vi "move.vi"() -> ()   [LabVIEW 2011]
uses:
  <vilib>/express/express arith-compare/Formula/XNode/ExpressFormulaBlockNode.xnode
panel:
  out "Obs":string
  in  "Boolean":bool
  out "Numero Impar":dbl
  in  "Generar NUmero Par 2":bool
  in  "Generar NUmero Par":bool
  out "Numero par":dbl
  # "Usando eventos generar un numero par al presionar un generar\npar y generar un impar al presionar un numero imprar"
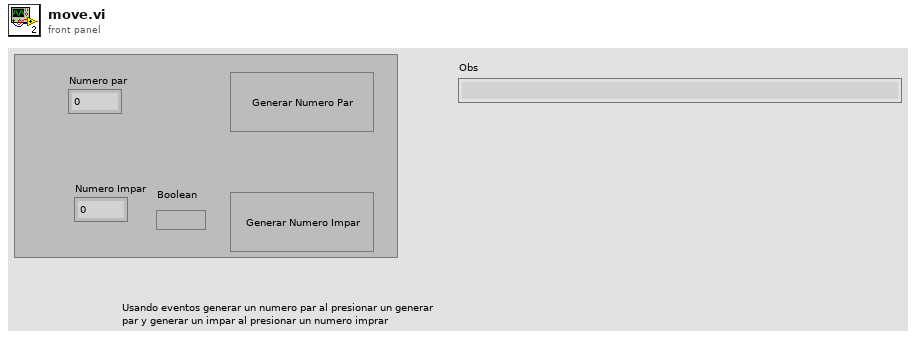
[diagram p1: front panel]
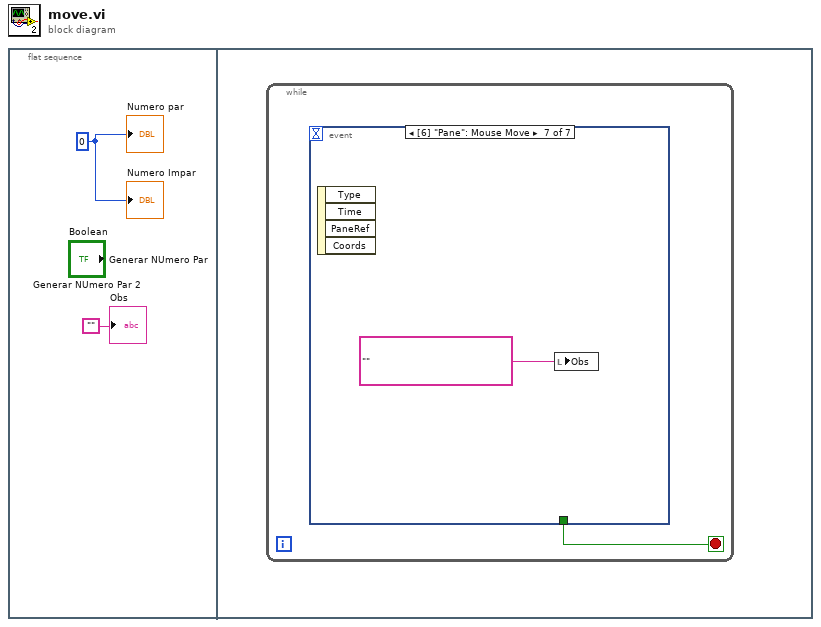
[diagram p0: block diagram]
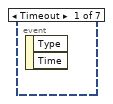
[diagram p2: hidden frame]
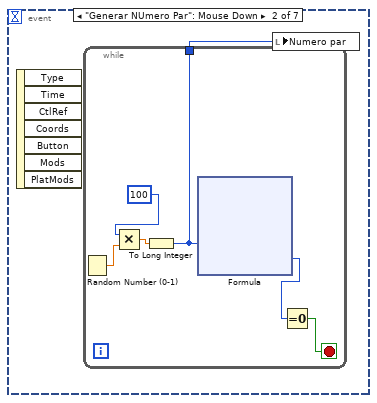
[diagram p3: hidden frame]
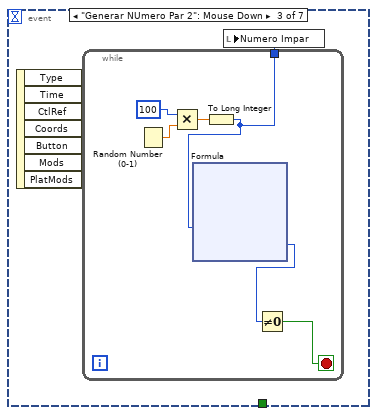
[diagram p4: hidden frame]
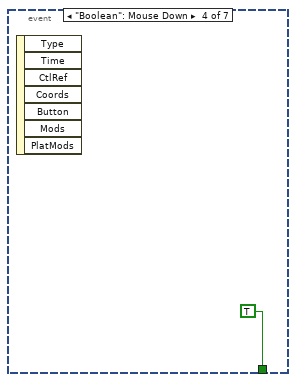
[diagram p5: hidden frame]
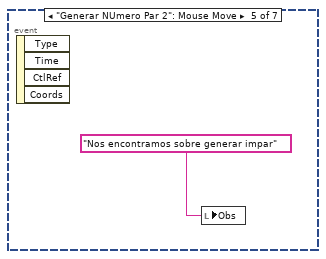
[diagram p6: hidden frame]
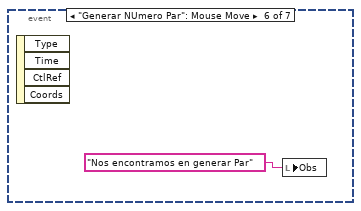
[diagram p7: hidden frame]
diagram:
  n1 = flat-sequence {
    frame #0 {
      w2 = 0
      "Numero par" <- w2
      "Numero Impar" <- w2
      "Obs" <- ""
    }
    frame #1 {
      n2 = while {
        stop <- w3 stop-if-true
        n3 = event shown="[6] \"Pane\": Mouse Move" {
          selector: _ -> [_ _ _ _ _ _ _]
          dyn-events: _ -> [_ _ _ _ _ _ _]
          timeout: _ -> [_ _ _ _ _ _ _]
          tunnel: [_ _ _ TRUE _ _ _] -> w3
          event Timeout {
            n4 = event-data() -> ()  [unwired: 1 in, 2 out]
          }
          event "Generar NUmero Par": Mouse Down {
            n5 = event-data() -> ()  [unwired: 1 in, 7 out]
            n6 = while {
              tunnel: [w5] -> w4
              stop <- w7 stop-if-true
              n7 = Random Number (0-1)() -> (number: 0 to 1=w8:dbl)
              n8 = Multiply(x=100, y=w8) -> (x*y=w10:dbl)
              n9 = To Long Integer(number=w10) -> (32bit integer=w5:i32)
              n10 = xnode "Formula"("X1"=w5) -> ("Result"=w6:i32)  [unwired: 1 in, 1 out]
              n11 = Equal To 0?(x=w6) -> (x = 0?=w7:bool)
            }
            n12 = local write "Numero par"(w4) -> ()
          }
          event "Generar NUmero Par 2": Mouse Down {
            n13 = event-data() -> ()  [unwired: 1 in, 7 out]
            n14 = while {
              tunnel: [w20] -> w19
              stop <- w22 stop-if-true
              n15 = Random Number (0-1)() -> (number: 0 to 1=w24:dbl)
              n16 = Multiply(x=100, y=w24) -> (x*y=w23:dbl)
              n17 = To Long Integer(number=w23) -> (32bit integer=w20:i32)
              n18 = xnode "Formula"("X1"=w20) -> ("Result"=w21:i32)  [unwired: 1 in, 1 out]
              n19 = Not Equal To 0?(x=w21) -> (x != 0?=w22:bool)
            }
            n20 = local write "Numero Impar"(w19) -> ()
          }
          event "Boolean": Mouse Down {
            n21 = event-data() -> ()  [unwired: 1 in, 7 out]
          }
          event "Generar NUmero Par 2": Mouse Move {
            n22 = event-data() -> ()  [unwired: 1 in, 4 out]
            n23 = local write "Obs"("Nos encontramos sobre generar impar") -> ()
          }
          event "Generar NUmero Par": Mouse Move {
            n24 = event-data() -> ()  [unwired: 1 in, 4 out]
            n25 = local write "Obs"("Nos encontramos en generar Par") -> ()
          }
          event Mouse Move {
            n26 = event-data() -> ()  [unwired: 1 in, 4 out]
            n27 = local write "Obs"("") -> ()
          }
        }
      }
    }
  }
